vi "Main.vi"() -> (0 "error out":errorcluster, 1 "Aborted":bool)   [LabVIEW 2024]
uses:
  LVMQTT-master/Controls/Connection_Return_Codes.ctl
  LVMQTT-master/Controls/QoS.ctl
  LVMQTT-master/Controls/Retain_Flag.ctl
  LVMQTT-master/Controls/DUP_Flag.ctl
  LVMQTT-master/Controls/Connect_Flags.ctl
  <vilib>/FPGAPlugInAG/cRIO-9068/niLvFpga_Open_cRIO-9068.vi
  <vilib>/rvi/interface/common/dynamic/niFpgaDynamicAddResources.vi
  <vilib>/rvi/interface/nirviOpenFPGA/nirviOpenFPGA.xnode
  FPGA Bitfiles/crio-9068-scan-t_FPGATarget_FPGAMAin_XA2NADVDmlU.lvbitx
  FPGA_MAin.vi
  LVMQTT-master/MQTT_Functions.lvlib
  <vilib>/NI_Real-Time Target Support.lvlib
panel:
  out "MessageID":i32
  out "Connection Status":T1=enum."Connection refused: not authorized"
  in  "Stop Publishing":bool
  out "Message":string
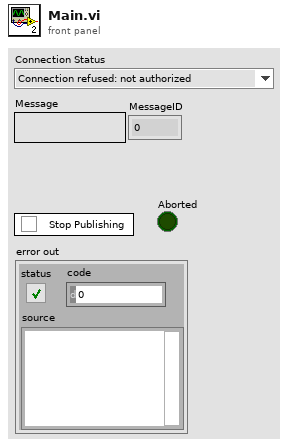
[diagram p1: front panel]
types:
  T1 = typedef "MQTT_Functions.lvlib/Connection_Return_Codes.ctl" = enum16{"Connection accepted", "Connection refused: unacceptable protocol version", "Connection refused: identifier rejected", "Connection refused: Server unavailable", "Connection refused: bad user name or password", "Connection refused: not authorized"}
  T2 = typedef "MQTT_Functions.lvlib/QoS.ctl" = enum8{"At most once", "At least once", "Exactly once", "Reserved"}
  T3 = typedef "MQTT_Functions.lvlib/DUP_Flag.ctl" = bool
  T4 = typedef "MQTT_Functions.lvlib/Retain_Flag.ctl" = bool
  T5 = cluster{"QoS":T2, "DUP":T3, "Retain":T4, "Keep Alive (sec)":u16}
  T6 = typedef "MQTT_Functions.lvlib/Connect_Flags.ctl" = cluster{"user name":bool, "password":bool, "will retain":bool, "will flag":bool, "clean session":bool, "reserved":bool, "will QoS":T2}
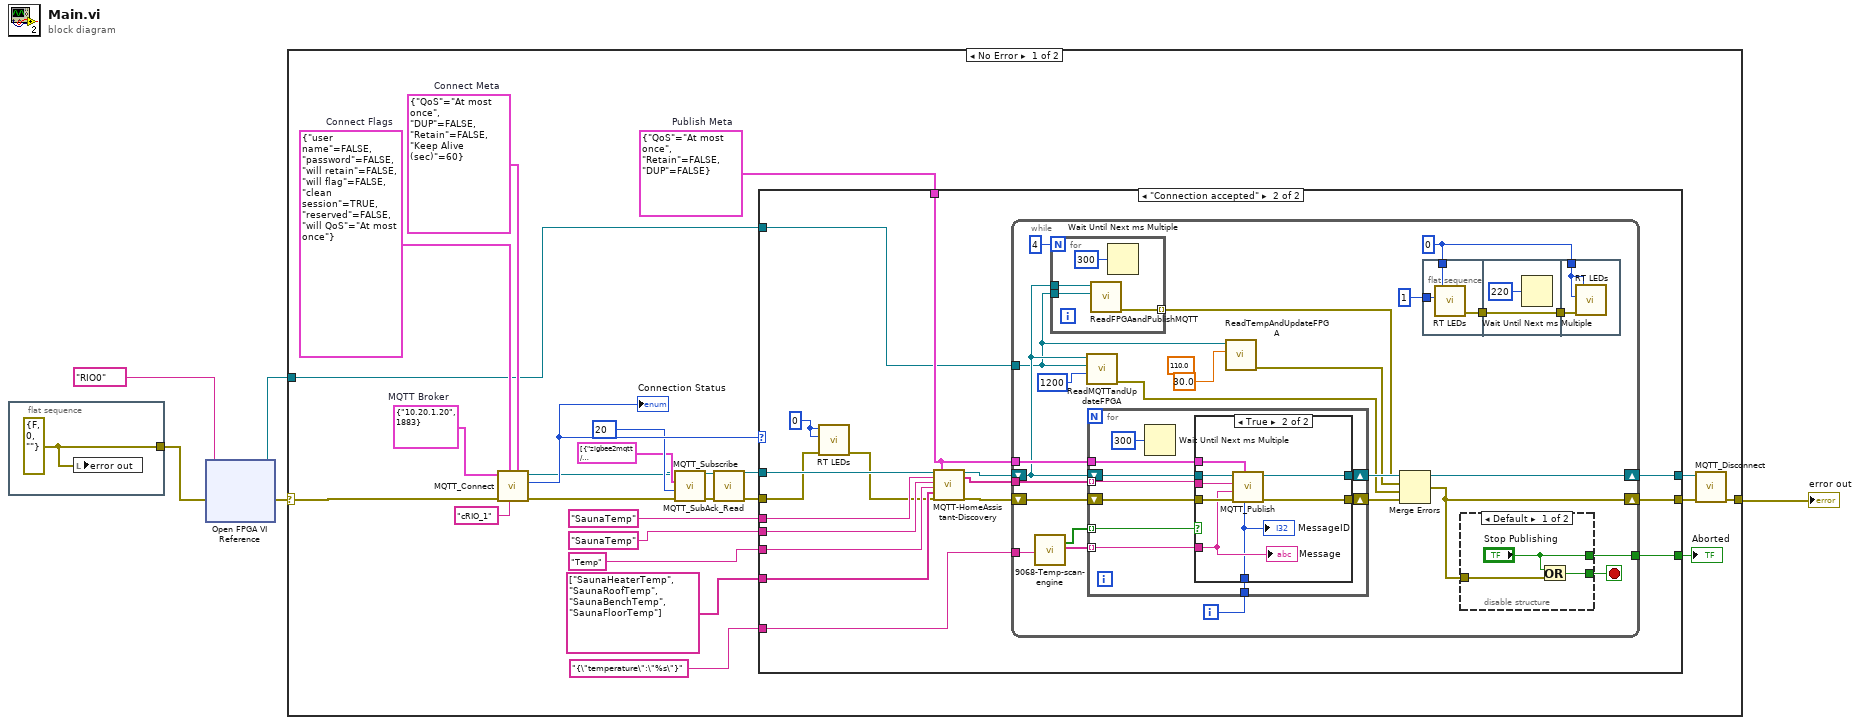
[diagram p0: block diagram]
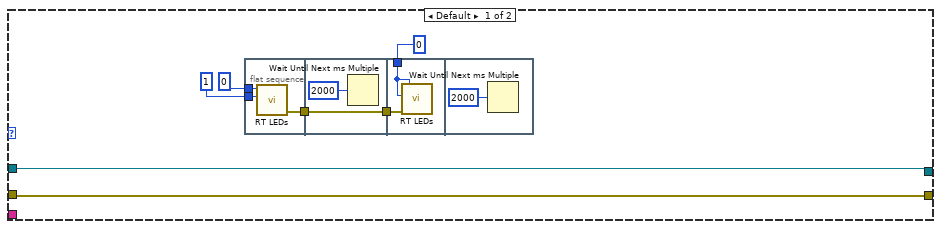
[diagram p2: hidden frame]
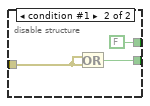
[diagram p3: hidden frame]
diagram:
  n1 = flat-sequence {
    tunnel: [w6] -> w3
    frame #0 {
      w6 = errorcluster {"status"=FALSE, "code"=0, "source"=""} ("error in (no error)")
      n2 = local write "error out"(w6) -> ()
    }
  }
  n3 = xnode "Open FPGA VI Reference"("error in"=w3, "resource name"=tag "RIO0") -> ("FPGA VI Reference Out"=w1:refnum<k20>, "error out"=w2:errorcluster)
  n4 = case shown="No Error" w2 {
    selector: w2 -> [w7 w125]
    tunnel: [w28 w125] -> w5
    tunnel: w1 -> [w8 _]
    frame No Error {
      w29 = T5 {"QoS"=enum."At most once", "DUP"=FALSE, "Retain"=FALSE, "Keep Alive (sec)"=60}  # Connect Meta
      w31 = T6 {"user name"=FALSE, "password"=FALSE, "will retain"=FALSE, "will flag"=FALSE, "clean session"=TRUE, "reserved"=FALSE, "will QoS"=enum."At most once"}  # Connect Flags
      w24 = cluster{"address (IP)":string, "port":u16} {"address (IP)"="10.20.1.20", "port"=1883}  # MQTT Broker
      w27 = cluster{"QoS":T2, "Retain":T4, "DUP":T3} {"QoS"=enum."At most once", "Retain"=FALSE, "DUP"=FALSE}  # Publish Meta
      n5 = call "MQTT_Connect.vi"("Connect Meta"=w29, "Client ID"="cRIO_1", "Connect Flags"=w31, "error in (no error)"=w7, "MQTT Broker"=w24) -> ("error out"=w10:errorcluster, "Connection Status"=w23:T1, "connection ID out"=w12:refnum<k5>)  [unwired: 4 in]
      "Connection Status" <- w23
      n6 = call "MQTT_Subscribe.vi"("error in (no error)"=w10, "Message ID"=u16 20, "Subscription Info Array"=cluster{"Topic":string, "QoS":T2}[] [{"Topic"="zigbee2mqtt/0xe0798dfffe57ec82", "QoS"=enum."At most once"}], "connection ID"=w12) -> ("error out"=w14:errorcluster, "connection ID out"=w15:refnum<k5>)  [unwired: 6 in]
      n7 = call "MQTT_SubAck_Read.vi"("error in (no error)"=w14, "connection ID"=w15) -> ("error out"=w9:errorcluster, "connection ID out"=w11:refnum<k5>)  [unwired: 7 in, 1 out]
      n8 = case shown="\"Connection accepted\"" w23 {
        tunnel: w27 -> [_ w56]
        tunnel: [w37 w63] -> w26
        tunnel: [w38 w62] -> w25
        tunnel: w9 -> [w37 w50]
        tunnel: w11 -> [w38 w61]
        tunnel: "{\"temperature\":\"%s\"}" ("Client ID") -> [_ w57]
        tunnel: string[] ["SaunaHeaterTemp", "SaunaRoofTemp", "SaunaBenchTemp", "SaunaFloorTemp"] ("ChannelNames") -> [_ w52]
        tunnel: "SaunaTemp" ("Device") -> [_ w55]
        tunnel: "SaunaTemp" ("DeviceName") -> [_ w54]
        tunnel: "Temp" ("ChannelBase") -> [_ w53]
        tunnel: [_ w48] -> w17
        tunnel: w8 -> [_ w47]
        frame Default {
          n9 = flat-sequence {
            tunnel: [w41] -> w36
            tunnel: 1 ("State") -> [w40]
            tunnel: 0 ("State") -> [w39]
            tunnel: w36 -> [w43]
            tunnel: [w43] -> w35
            tunnel: w35 -> [w45]
            tunnel: 0 ("State") -> [w44]
            frame #0 {
              n10 = call <vilib>:"RT LEDs.vi"("State"=w40, "LED Num"=w39) -> ("error out"=w41:errorcluster)  [unwired: 4 in, 1 out]
            }
            frame #1 {
              n11 = Wait Until Next ms Multiple(millisecond multiple=u32 2000) -> ()  [unwired: 1 out]
            }
            frame #2 {
              n12 = call <vilib>:"RT LEDs.vi"("error in (no error)"=w45, "State"=w44, "LED Num"=w44) -> ()  [unwired: 3 in, 2 out]
            }
            frame #3 {
              n13 = Wait Until Next ms Multiple(millisecond multiple=u32 2000) -> ()  [unwired: 1 out]
            }
          }
        }
        frame "Connection accepted" {
          w49 = 0 ("State")
          n14 = call <vilib>:"RT LEDs.vi"("error in (no error)"=w50, "State"=w49, "LED Num"=w49) -> ("error out"=w51:errorcluster)  [unwired: 3 in, 1 out]
          n15 = call "MQTT-HomeAssistant-Discovery.vi"("TCP Network Connection in"=w61, "Device"=w55, "DeviceName"=w54, "ChannelBase"=w53, "ChannelNames"=w52, "error in (no error)"=w51, "Publish Meta"=w56) -> ("TCP Network Connection out"=w59:refnum<k5>, "Topics"=w58:string[], "error out"=w60:errorcluster)  [unwired: 10 in]
          n16 = while {
            tunnel: w56 -> [w86]
            shift-right: [w72] -> w63
            shift-left: w60 -> [w87]
            shift-right: [w85] -> w62
            shift-left: w59 -> [w68]
            tunnel: w58 -> [w79]
            tunnel: w57 -> [w78]
            tunnel: [w74] -> w48
            tunnel: w47 -> [w67]
            i -> [w80]
            stop <- w84 stop-if-true
            (unwired) 110.0 ("TempThreshold")
            w73 = 0 ("State")
            n17 = call "9068-Temp-scan-engine.vi"("MessageFormat"=w78) -> ("updated?"=w82:bool[], "Messages"=w81:string[])  [unwired: 16 in, 1 out]
            n18 = for {
              N: 4 -> [_]
              tunnel: w68 -> [w90]
              tunnel: w67 -> [w89]
              tunnel: [w88] -> w66 mode=indexing
              n19 = call "ReadFPGAandPublishMQTT.vi"("FPGA VI Reference"=w89, "MQTT"=w90) -> ("error out"=w88:errorcluster)  [unwired: 8 in, 1 out]
              n20 = Wait Until Next ms Multiple(millisecond multiple=u32 300) -> ()  [unwired: 1 out]
            }
            n21 = call "ReadMQTTandUpdateFPGA.vi"("timeout ms (25000)"=1200, "FPGA VI Reference"=w67, "MQTT"=w68) -> ("error out"=w71:errorcluster)  [unwired: 8 in]
            n22 = for {
              tunnel: w86 -> [w112]
              tunnel: w82 -> [w109] mode=indexing
              shift-right: [w111] -> w85
              shift-left: w68 -> [w114]
              shift-right: [w110] -> w83
              shift-left: w87 -> [w113]
              tunnel: w81 -> [w108] mode=indexing
              tunnel: w80 -> [w106]
              tunnel: w79 -> [w105] mode=indexing
              n23 = Wait Until Next ms Multiple(millisecond multiple=u32 300) -> ()  [unwired: 1 out]
              n24 = case shown="True" w109 {
                tunnel: w105 -> [_ w124]
                tunnel: w114 -> [w116 w123]
                tunnel: w113 -> [w115 w122]
                tunnel: w112 -> [_ w121]
                tunnel: [w116 w120] -> w111
                tunnel: [w115 w119] -> w110
                tunnel: w108 -> [_ w118]
                tunnel: w106 -> [_ w117]
                frame False {
                }
                frame True {
                  n25 = call "MQTT_Publish.vi"("Message ID"=w117, "Publish Meta"=w121, "error in (no error)"=w122, "Message to be published"=w118, "Topic"=w124, "connection ID"=w123) -> ("error out"=w119:errorcluster, "connection ID out"=w120:refnum<k5>)  [unwired: 4 in]
                  "Message" <- w118
                  "MessageID" <- w117
                }
              }
            }
            n26 = call "ReadTempAndUpdateFPGA.vi"("TempThreshold"=30.0, "FPGA VI Reference"=w67) -> ("error out"=w65:errorcluster)  [unwired: 9 in]
            n27 = Merge Errors(w66, w65, w71, w83) -> (w72:errorcluster)
            n28 = flat-sequence {
              tunnel: [w94] -> w77
              tunnel: 1 ("State") -> [w93]
              tunnel: w73 -> [w92]
              tunnel: w77 -> [w96]
              tunnel: [w96] -> w76
              tunnel: w76 -> [w98]
              tunnel: w73 -> [w97]
              frame #0 {
                n29 = call <vilib>:"RT LEDs.vi"("State"=w93, "LED Num"=w92) -> ("error out"=w94:errorcluster)  [unwired: 4 in, 1 out]
              }
              frame #1 {
                n30 = Wait Until Next ms Multiple(millisecond multiple=u32 220) -> ()  [unwired: 1 out]
              }
              frame #2 {
                n31 = call <vilib>:"RT LEDs.vi"("error in (no error)"=w98, "State"=w97, "LED Num"=w97) -> ()  [unwired: 3 in, 2 out]
              }
            }
            n32 = disable-structure shown="Default" {
              disable-tunnel: [w101 w104] -> w84
              disable-tunnel: w72 -> [w100 w103]
              disable-tunnel: ["Stop Publishing" FALSE ("Stop Publishing")] -> w74
              frame condition #0 (active) {
                n33 = Or(x="Stop Publishing", y=w100) -> (x .or. y?=w101:bool)
              }
              frame condition #1 {
                n34 = Or(x=w103, y=w103) -> (x .or. y?=w104:bool)
              }
            }
          }
        }
      }
      "Aborted" <- w17
      n35 = call "MQTT_Disconnect.vi"("error in (no error)"=w26, "connection ID"=w25) -> ("error out"=w28:errorcluster)  [unwired: 9 in]
    }
    frame Error {
    }
  }
  "error out" <- w5
